vi "NovaTech409A_Init.vi"(2 "error in (no error)":errorcluster, 3 "Set Phase (F)?":bool, 4 "VISA resource name":refnum<visa-resource-name>="COM1") -> (0 "error out":errorcluster, 1 "VISA resource name out":refnum<visa-resource-name>="COM1")   [LabVIEW 2013, in "Novatech 409A.lvlib"]
uses:
  Novatech 409A.lvlib
  <vilib>/Instr/_visa.llb/VISA Configure Serial Port (Instr).vi
panel:
  out "read buffer 2":string="OK\r\n"
  out "read buffer 1":string="OK\r\n"
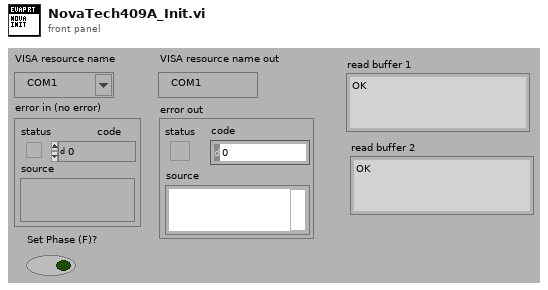
[diagram p1: front panel]
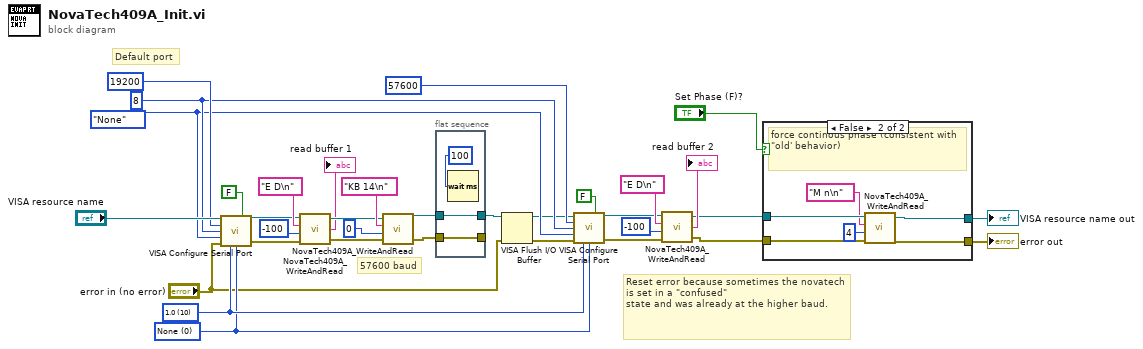
[diagram p0: block diagram]
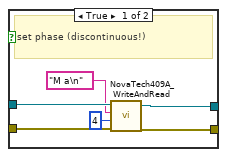
[diagram p2: hidden frame]
diagram:
  w18 = u16 0 items=["None", "XON/XOFF", "RTS/CTS", "XON/XOFF & RTS/CTS", "DTR/DSR", "XON/XOFF & DTR/DSR"] ("flow control (0:none)")
  w19 = u16 10 items=["1.0"=10, "1.5"=15, "2.0"=20] ("stop bits (10: 1 bit)")
  w20 = enum16{"None", "Odd", "Even", "Mark", "Space"}."None" ("parity (0:none)")
  w21 = u16 8 ("data bits (8)")
  # "Reset error because sometimes the novatech is set in a \"confused\"\nstate and was already at the higher baud."
  # "57600 baud"
  # "Default port"
  n1 = call-poly "VISA Configure Serial Port"("VISA resource name"="VISA resource name", "Enable Termination\nChar (T)"=FALSE ("Enable Termination\nChar (T)"), "baud rate (9600)"=u32 19200, "data bits (8)"=w21, "parity (0:none)"=w20, "error in (no error)"="error in (no error)", "stop bits (10: 1 bit)"=w19, "flow control (0:none)"=w18) -> ("VISA resource name out"=w29:refnum<visa-resource-name>, "error out"=w28:errorcluster)  [unwired: 6 out]
  n2 = call "NovaTech409A_WriteAndRead.vi"("error in (no error)"=w28, "Number of Bytes"=-100, "write buffer"="E D\n", "VISA resource name"=w29) -> ("error out"=w25:errorcluster, "read buffer"=→"read buffer 1":string, "VISA resource name out"=w24:refnum<visa-resource-name>)
  n3 = call "NovaTech409A_WriteAndRead.vi"("error in (no error)"=w25, "Number of Bytes"=0, "write buffer"="KB 14\n", "VISA resource name"=w24) -> ("error out"=w13:errorcluster, "VISA resource name out"=w14:refnum<visa-resource-name>)  [unwired: 1 out]
  n4 = flat-sequence {
    tunnel: [w37] -> w12
    tunnel: w14 -> [w37]
    tunnel: w13 -> [w36]
    tunnel: [w36] -> _
    frame #0 {
      n5 = Wait (ms)(milliseconds to wait=u32 100 ("baud rate (9600)")) -> ()  [unwired: 1 out]
    }
  }
  n6 = VISA Flush I/O Buffer(VISA resource name=w12, error in (no error)="error in (no error)") -> (VISA resource name out=w16:refnum<visa-resource-name>, error out=w15:errorcluster)  [unwired: 1 out]
  n7 = call-poly "VISA Configure Serial Port"("VISA resource name"=w16, "Enable Termination\nChar (T)"=FALSE ("Enable Termination\nChar (T)"), "baud rate (9600)"=u32 57600, "data bits (8)"=w21, "parity (0:none)"=w20, "error in (no error)"=w15, "stop bits (10: 1 bit)"=w19, "flow control (0:none)"=w18) -> ("VISA resource name out"=w8:refnum<visa-resource-name>, "error out"=w7:errorcluster)  [unwired: 1 in, 5 out]
  n8 = call "NovaTech409A_WriteAndRead.vi"("error in (no error)"=w7, "Number of Bytes"=-100, "write buffer"="E D\n", "VISA resource name"=w8) -> ("error out"=w3:errorcluster, "read buffer"=→"read buffer 2":string, "VISA resource name out"=w5:refnum<visa-resource-name>)
  n9 = case shown="False" "Set Phase (F)?" {
    tunnel: w5 -> [w43 w49]
    tunnel: [w42 w48] -> w4
    tunnel: w3 -> [w41 w47]
    tunnel: [w40 w46] -> w2
    frame True {
      # "set phase (discontinuous!)"
      n10 = call "NovaTech409A_WriteAndRead.vi"("error in (no error)"=w41, "Number of Bytes"=4, "write buffer"="M a\n", "VISA resource name"=w43) -> ("error out"=w40:errorcluster, "VISA resource name out"=w42:refnum<visa-resource-name>)  [unwired: 1 out]
    }
    frame False {
      # "force continous phase (consistent with \"old' behavior)"
      n11 = call "NovaTech409A_WriteAndRead.vi"("error in (no error)"=w47, "Number of Bytes"=4, "write buffer"="M n\n", "VISA resource name"=w49) -> ("error out"=w46:errorcluster, "VISA resource name out"=w48:refnum<visa-resource-name>)  [unwired: 1 out]
    }
  }
  "error out" <- w2
  "VISA resource name out" <- w4
